vi "Queue.vi"(0 "Element_In":dbl, 9 "Operation":T1=enum."Enqueue", 11 "Error_In":errorcluster) -> (3 "Overflow":bool, 4 "Element_Out":dbl, 6 "Sum":dbl, 14 "Underflow":bool, 15 "Error_Out":errorcluster)   [LabVIEW 2021]
doc: "This is a LV2, Which has array as its storage unit. hence can be used as queue. it is provided with the pins as follows\nElement_in - Data to be Enqueued\nElement_out - Data Dequeued\nSum - Provides the total sum of elelments in the queue\noverflow and underflow - flags that turns on when overflow and underflow conditions accours.\nError_in and Error_out where given for Error handling"
uses:
  Type_Def/Size_Pointer.ctl
  Type_Def/Operation_Queue.ctl
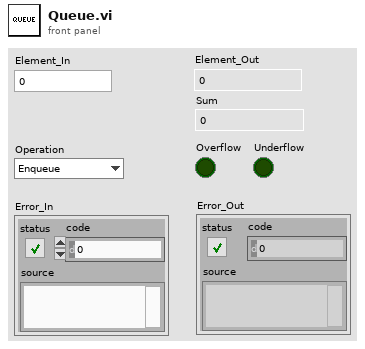
[diagram p1: front panel]
types:
  T1 = typedef "Operation_Queue.ctl" = enum16{"Initialize", "Enqueue", "Dequeue", "Sum"}
  T2 = typedef "Size_Pointer.ctl" = cluster{"Head_Pointer":i64, "Dimension_Size (10)":i64, "Queue":dbl[]}
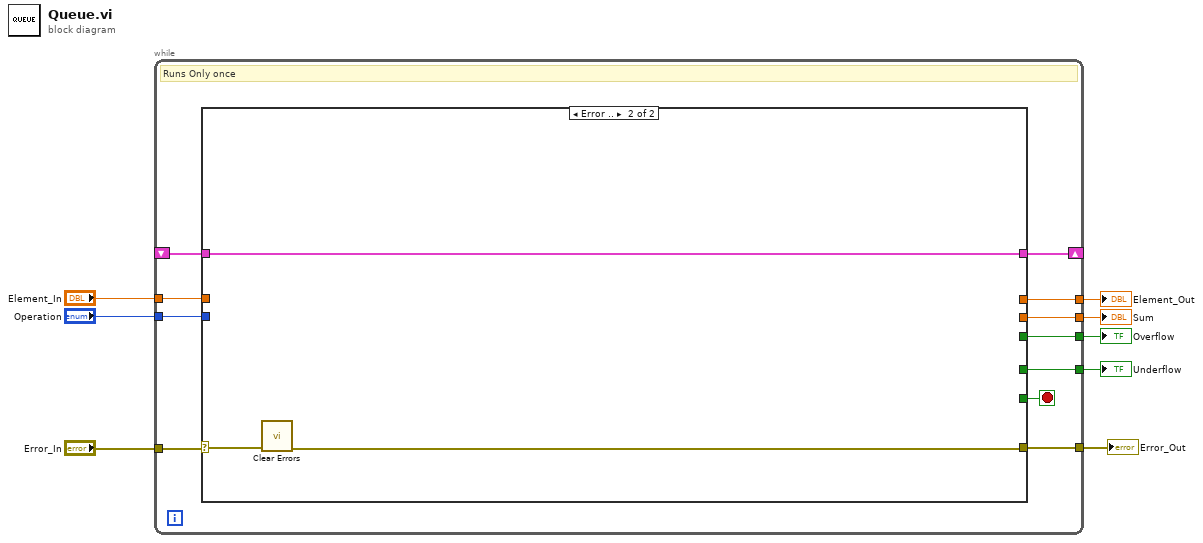
[diagram p0: block diagram]
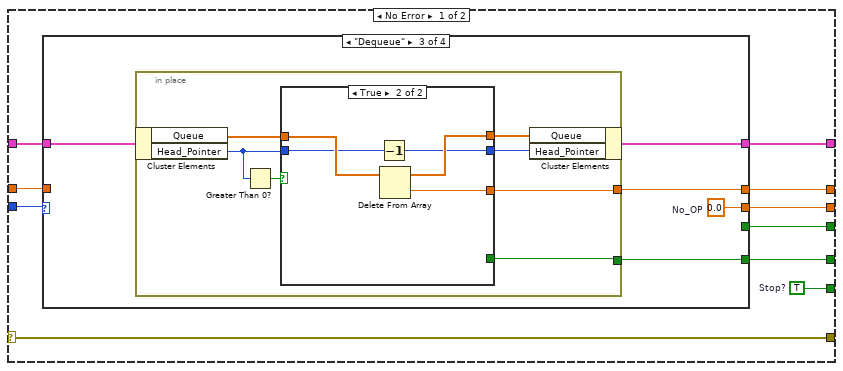
[diagram p2: hidden frame]
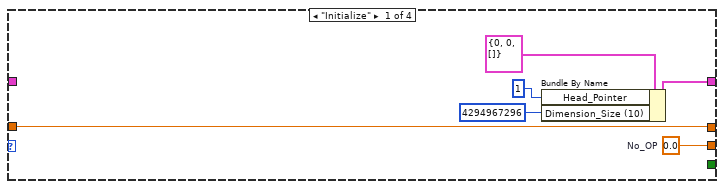
[diagram p3: hidden frame]
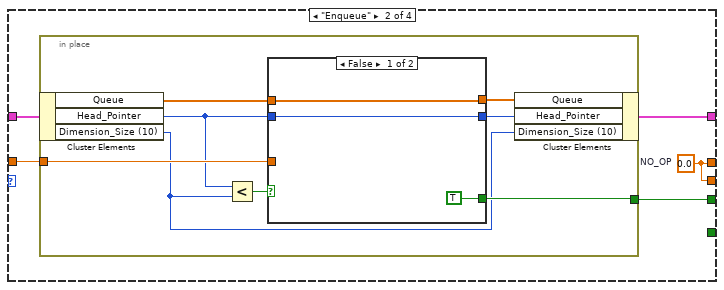
[diagram p4: hidden frame]
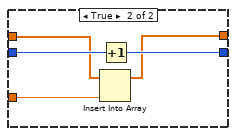
[diagram p5: hidden frame]
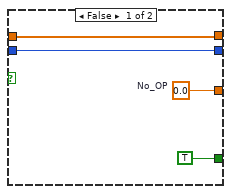
[diagram p6: hidden frame]
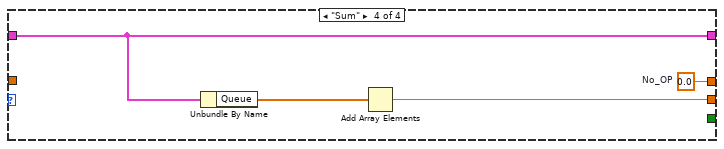
[diagram p7: hidden frame]
diagram:
  n1 = while {
    tunnel: [w19] -> w8
    tunnel: [w18] -> w7
    tunnel: "Element_In" -> [w17]
    tunnel: "Operation" -> [w16]
    tunnel: [w14] -> w4
    tunnel: [w13] -> w3
    shift-right: [w12] -> _
    shift-left: _ -> [w11]
    tunnel: "Error_In" -> [w10]
    tunnel: [w9] -> w1
    stop <- w15 stop-if-true
    # "Runs Only once"
    n2 = case shown="Error .." w10 {
      selector: w10 -> [w20 w84]
      tunnel: [w29 _] -> w19
      tunnel: [w28 _] -> w18
      tunnel: w17 -> [w27 _]
      tunnel: w16 -> [w26 _]
      tunnel: [w25 _] -> w15
      tunnel: [w24 _] -> w14
      tunnel: [w23 _] -> w13
      tunnel: [w22 w83] -> w12
      tunnel: w11 -> [w21 w83]
      tunnel: [w20 w82] -> w9
      frame No Error {
        w25 = TRUE  # Stop?
        n3 = case shown="\"Dequeue\"" w26 {
          tunnel: w21 -> [_ w37 w57 w80]
          tunnel: w27 -> [w34 w40 _ _]
          tunnel: [w34 w38 w61 w81] -> w29
          tunnel: [w35 w38 w60 w79] -> w28
          tunnel: [_ w39 _ _] -> w24
          tunnel: [_ _ w59 _] -> w23
          tunnel: [w32 w36 w58 w80] -> w22
          frame "Initialize" {
            w35 = 0.0  # No_OP
            n4 = Bundle By Name(cluster=T2 {"Head_Pointer"=0, "Dimension_Size (10)"=0, "Queue"=[]} ("Queue_and_Pointer"), "Head_Pointer"=i64 1 ("Dimension_Size (10)"), "Dimension_Size (10)"=i64 4294967296) -> (w32:T2)
          }
          frame "Enqueue" {
            w38 = 0.0  # NO_OP
            n5 = in-place "In Place Element Structure" {
              in-place-border: w40 -> [w48]
              in-place-border: [w46] -> w39
              n6 = in-place-cluster #1(w37) -> ("Queue"=w45:dbl[], "Head_Pointer"=w42:i64, "Dimension_Size (10)"=w41:i64)
              n7 = Less?(x=w42, y=w41) -> (x < y?=w47:bool)
              n8 = case shown="False" w47 {
                tunnel: w48 -> [_ w53]
                tunnel: w45 -> [w50 w52]
                tunnel: [w50 w54] -> w43
                tunnel: w42 -> [w51 w56]
                tunnel: [w51 w55] -> w44
                tunnel: [TRUE _] -> w46
                frame False {
                }
                frame True {
                  n9 = Insert Into Array(array=w52, new element=w53) -> (w54:dbl[])  [unwired: 1 in]
                  n10 = Increment(x=w56) -> (x+1=w55:i64)
                }
              }
              n11 = in-place-cluster #1("Queue"=w43, "Head_Pointer"=w44, "Dimension_Size (10)"=w41) -> (w36:T2)
            }
          }
          frame "Dequeue" {
            w60 = 0.0  # No_OP
            n12 = in-place "In Place Element Structure" {
              in-place-border: [w68] -> w61
              in-place-border: [w66] -> w59
              n13 = in-place-cluster #2(w57) -> ("Queue"=w63:dbl[], "Head_Pointer"=w64:i64)
              n14 = Greater Than 0?(x=w64) -> (x > 0?=w65:bool)
              n15 = case shown="True" w65 {
                tunnel: [w72 w76] -> w62
                tunnel: w63 -> [w72 w77]
                tunnel: [w70 w75] -> w68
                tunnel: w64 -> [w71 w74]
                tunnel: [w71 w73] -> w67
                tunnel: [TRUE _] -> w66
                frame False {
                  w70 = 0.0  # No_OP
                }
                frame True {
                  n16 = Decrement(x=w74) -> (x-1=w73:i64)
                  n17 = Delete From Array(array=w77) -> (deleted portion=w75:dbl, array with subset deleted=w76:dbl[])  [unwired: 2 in]
                }
              }
              n18 = in-place-cluster #2("Queue"=w62, "Head_Pointer"=w67) -> (w58:T2)
            }
          }
          frame "Sum" {
            w81 = 0.0  # No_OP
            n19 = Unbundle By Name(w80) -> ("Queue"=w78:dbl[])
            n20 = Add Array Elements(numeric array=w78) -> (sum=w79:dbl)
          }
        }
      }
      frame Error {
        n21 = call <vilib>:"Clear Errors.vi"("error in (no error)"=w84) -> ("error out"=w82:errorcluster)  [unwired: 5 in, 1 out]
      }
    }
  }
  "Error_Out" <- w1
  "Element_Out" <- w8
  "Sum" <- w7
  "Overflow" <- w4
  "Underflow" <- w3
